vi "Chop Integration Bins.vi"(4 "tolerance":dbl=1e-10, 6 "variable output":string, 7 "variable input":string, 8 "error in (no error)":errorcluster, 9 "formula":string, 10 "Chop In":bool[](array[boolean]), 11 "Bins In":cluster{"lower limit":dbl, "upper limit":dbl}[](array[cluster])) -> (0 "error out":errorcluster, 2 "Chop Out":bool[](array[boolean]), 3 "Bins Out":cluster{"lower limit":dbl, "upper limit":dbl}[](array[cluster]))   [LabVIEW 2020, in "NI_AALPro.lvlib"]
uses:
  <vilib>/Analysis/NI_AALPro.lvlib
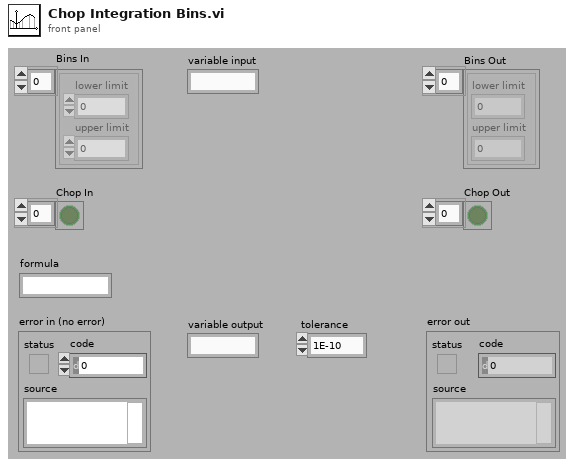
[diagram p1: front panel]
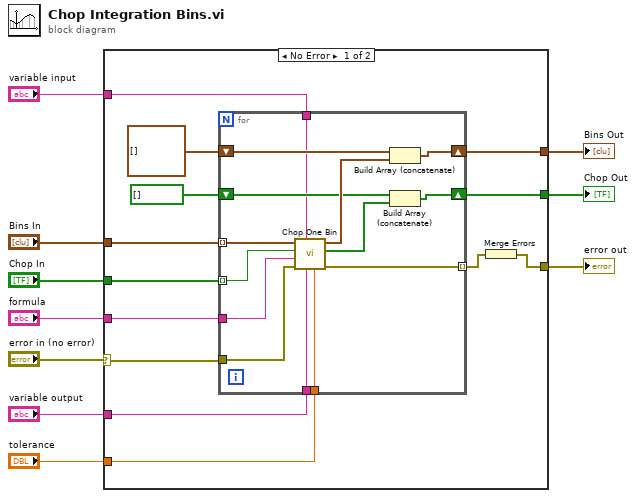
[diagram p0: block diagram]
diagram:
  n1 = case shown="No Error" "error in (no error)" {
    selector: "error in (no error)" -> [w13 w38]
    tunnel: "Bins In" -> [w23 _]
    tunnel: "formula" -> [w22 _]
    tunnel: "variable output" -> [w21 _]
    tunnel: [w19 _] -> w7
    tunnel: "Chop In" -> [w17 _]
    tunnel: [w16 _] -> w5
    tunnel: "variable input" -> [w15 _]
    tunnel: [w11 w38] -> w3
    tunnel: "tolerance" -> [w14 _]
    frame No Error {
      n2 = for {
        tunnel: w23 -> [w36] mode=indexing
        tunnel: w22 -> [w29]
        tunnel: w21 -> [w28]
        shift-right: [w32] -> w19
        shift-left: cluster{dbl, dbl}[] [] -> [w33]
        shift-right: [w37] -> w16
        shift-left: bool[] [] -> [w30]
        tunnel: w17 -> [w35] mode=indexing
        tunnel: w15 -> [w27]
        tunnel: [w26] -> w12 mode=indexing
        tunnel: w14 -> [w25]
        tunnel: w13 -> [w24]
        n3 = call <vilib>:"Chop One Bin.vi"("tolerance"=w25, "variable output"=w28, "variable input"=w27, "error in (no error)"=w24, "formula"=w29, "chop?"=w35, "bin"=w36) -> ("error out"=w26:errorcluster, "Chop Out"=w31:bool[], "Bins Out"=w34:cluster{"lower limit":dbl, "upper limit":dbl}[])  [unwired: 2 in]
        n4 = Build Array (concatenate)(w33, w34) -> (w32:cluster{"lower limit":dbl, "upper limit":dbl}[])
        n5 = Build Array (concatenate)(w30, w31) -> (w37:bool[])
      }
      n6 = Merge Errors(w12) -> (w11:errorcluster)
    }
    frame Error {
    }
  }
  "Bins Out" <- w7
  "Chop Out" <- w5
  "error out" <- w3
